vi "testtoxmlandbacktest.vi"() -> ()   [LabVIEW 2013, in "VI-Test.lvlib"]
uses:
  lib/VI-Test.lvlib
  classes/Tests/TestInterface/TestInterface.lvclass
  classes/Devices/emTestCWS500N/EMTestCWS500N.lvclass
  lib/DataCreation.lvlib
panel:
  out "Tests":refnum<class "TestInterface.lvclass">[](array[class])
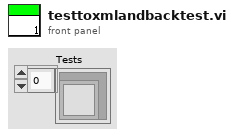
[diagram p1: front panel]
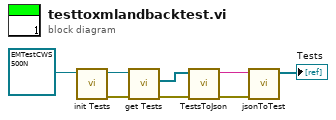
[diagram p0: block diagram]
diagram:
  n1 = call-dynamic "init Tests.vi"("EMTestCWS500N Eingang"=refnum<class "EMTestCWS500N.lvclass"> refnum) -> ("error out"=w4:errorcluster, "EMTestCWS500N Ausgang"=w5:refnum<class "EMTestCWS500N.lvclass">)  [unwired: 9 in]
  n2 = call-dynamic "get Tests.vi"("error in (no error)"=w4, "DeviceInterface (Eingang)"=w5) -> ("error out"=w3:errorcluster, "Tests"=w2:refnum<class "TestInterface.lvclass">[])  [unwired: 7 in, 1 out]
  n3 = call "TestsToJson.vi"("error in (no error)"=w3, "Test Array"=w2) -> ("error out"=w7:errorcluster, "JSON string"=w8:string)  [unwired: 8 in]
  n4 = call "jsonToTest.vi"("error in (no error)"=w7, "JSON string"=w8) -> ("Tests"=→"Tests":refnum<class "TestInterface.lvclass">[])  [unwired: 8 in, 1 out]
